vi "Format Library List Table.vi"(5 "Detail Level":T1, 7 "Msg Chain in":string, 8 "error in (no error)":errorcluster, 10 "Library Info Array":T2[](array[typedef]), 11 "VIDoc Printer - Confluence In":refnum<class "VIDoc Printer - Confluence.lvclass">) -> (0 "error out":errorcluster, 2 "Table Text":string, 3 "VIDoc Printer - Confluence Out":refnum<class "VIDoc Printer - Confluence.lvclass">)   [LabVIEW 2023, in "VIDoc Printer - Confluence.lvlib" / "VIDoc Printer - Confluence.lvclass"]
uses:
  VIDoc Printer - Confluence.lvclass
  C:/projects/DMC/Tooling/Git-Action-Service/Source/Documentation Generation/Printers/Printer/VIDoc Printer.lvclass
  Parsing/TypeDefs/Base Library Info Cluster.ctl
  <vilib>/picture/picture.llb/imagedata.ctl
  Settings/Printer Settings/Detail Level Enum.ctl
  VIDoc Printer - Confluence.lvclass/VIDoc Printer - Confluence.ctl
  Accessors/Get Library Column Ordering - Full.vi
  Accessors/Get Library Column Ordering - Minimal.vi
  Accessors/Get Library Column Ordering - Standard.vi
  Accessors/Get Sortable Tables.vi
  Printer/VIDoc Printer.lvclass
  UI Interaction/UI Interaction.lvclass
  Confluence Formatting/Confluence Formatting.lvlib
  C:/projects/DMC/Tooling/Git-Action-Service/Source/Documentation Generation/Printers/Confluence Printer/VIDoc Printer - Confluence.lvclass
  Parsing/VIDoc Parsing.lvlib
  Settings/Printer Settings/Printer Settings.lvclass
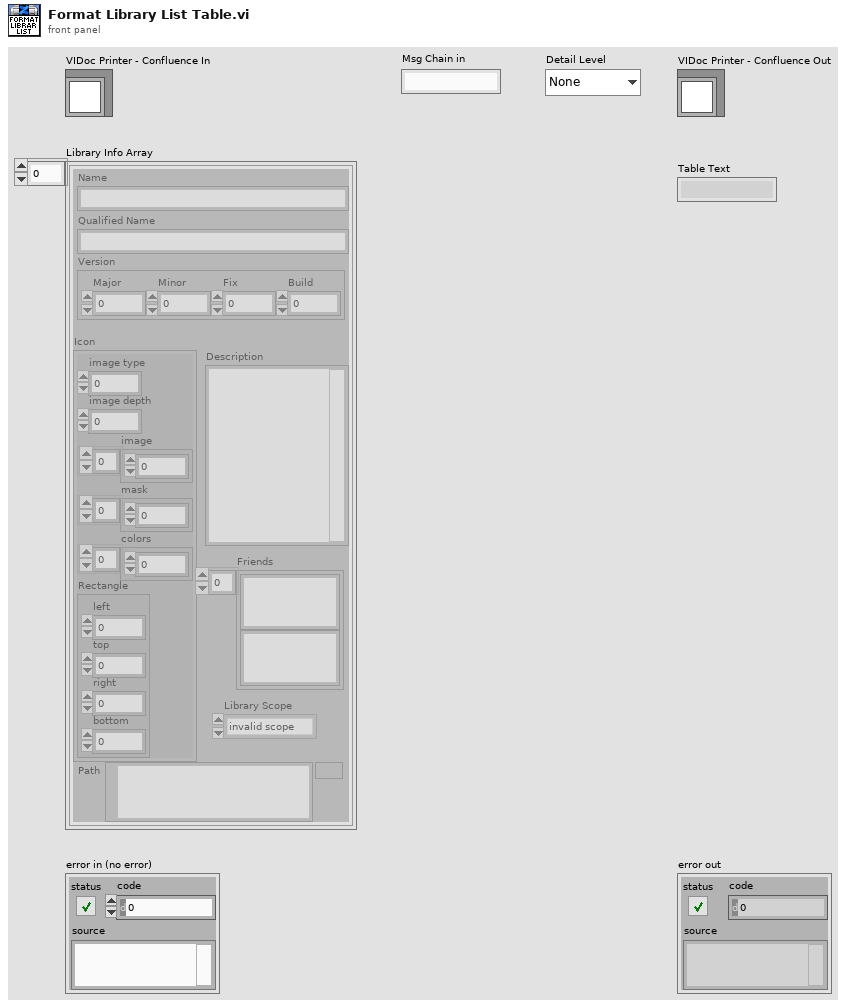
[diagram p1: front panel]
types:
  T1 = typedef "VIDoc Printer.lvlib/Printer Settings.lvclass/Detail Level Enum.ctl" = enum16{"None", "Minimal", "Standard", "Full"}
  T2 = typedef "VIDoc Parsing.lvlib/Base Library Info Cluster.ctl" = cluster{"Name":string, "Icon":T3, "Version":cluster{"Major":u16, "Minor":u16, "Fix":u16, "Build":u16}, "Description":string, "Path":path, "Friends":string[], "Library Scope":enum32{"invalid scope", "public", "private", "protected", "community"}, "Qualified Name":string}
  T3 = typedef "imagedata.ctl" = cluster{"image type":i32, "image depth":i32, "image":u8[], "mask":u8[], "colors":u32[], "Rectangle":cluster{"left":i16, "top":i16, "right":i16, "bottom":i16}}
  T4 = cluster{"Major":u16, "Minor":u16, "Fix":u16, "Build":u16}
  T5 = typedef "VIDoc Printer - Confluence.lvlib/VIDoc Settings - Confluence.lvclass/Class Info Column.ctl" = enum16{"Image", "Name", "Description", "Version", "Last Change", "Author", "Commit Hash", "Branch", "Qualified Name", "TransferMustOverrides", "ChildRefsRestricted"}
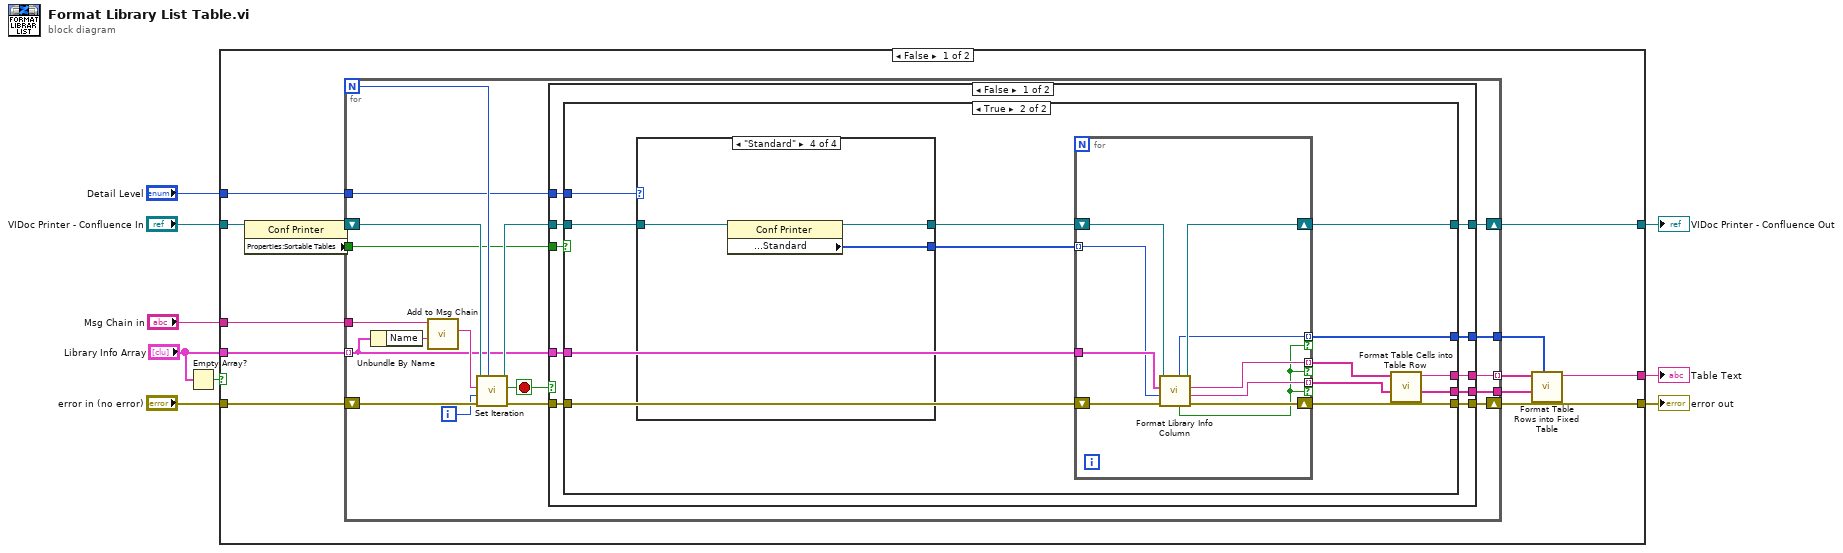
[diagram p0: block diagram]
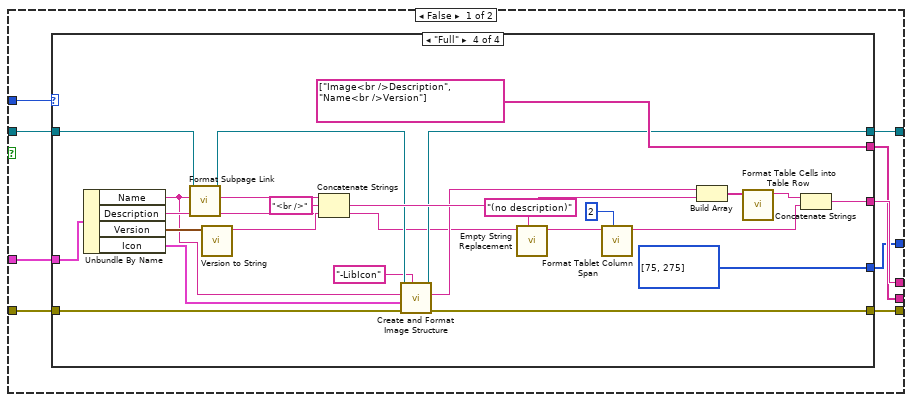
[diagram p2: hidden frame]
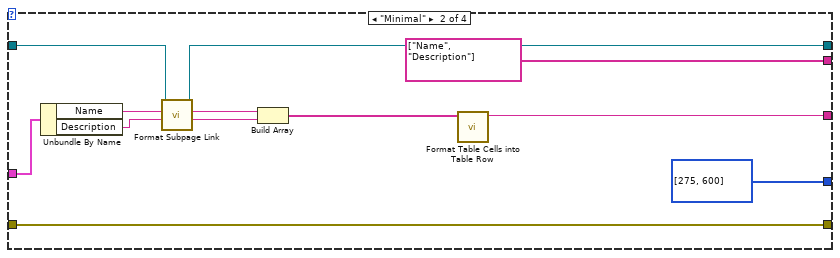
[diagram p4: hidden frame]
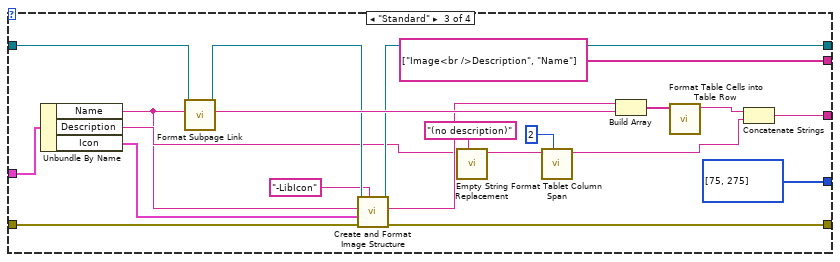
[diagram p5: hidden frame]
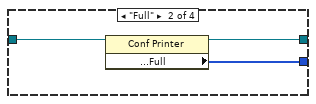
[diagram p7: hidden frame]
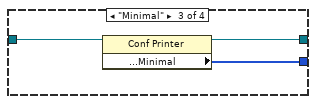
[diagram p8: hidden frame]
diagram:
  n1 = Empty Array?(array="Library Info Array") -> (empty?=w5:bool)
  n2 = case shown="False" w5 {
    tunnel: [w22 w153] -> w9
    tunnel: [w13 _] -> w8
    tunnel: [w21 w154] -> w7
    tunnel: "VIDoc Printer - Confluence In" -> [w17 w154]
    tunnel: "error in (no error)" -> [w20 w153]
    tunnel: "Library Info Array" -> [w19 _]
    tunnel: "Msg Chain in" -> [w18 _]
    tunnel: "Detail Level" -> [w16 _]
    frame False {
      n3 = property class="Conf Printer"(reference=w17) -> (reference out=w11:refnum<class "VIDoc Printer - Confluence.lvclass">, "Properties:Sortable Tables"=w10:bool)  [unwired: 1 in, 1 out]
      n4 = for {
        N -> [w38]
        shift-right: [w29] -> w22
        shift-left: w20 -> [w40]
        shift-right: [w31] -> w21
        shift-left: w11 -> [w39]
        tunnel: w19 -> [w26] mode=indexing
        tunnel: w18 -> [w34]
        tunnel: w16 -> [w30]
        tunnel: [w28] -> w15 mode=indexing
        tunnel: [w27] -> w14
        tunnel: [w25] -> w12
        tunnel: w10 -> [w23]
        i -> [w37]
        stop <- w24 stop-if-true
        n5 = Unbundle By Name(w26) -> ("Name"=w36:string)
        n6 = call "Add to Msg Chain.vi"("New"=w36, "Msg Chain in"=w34) -> ("Msg Chain out"=w35:string)  [unwired: 9 in]
        n7 = call "Set Iteration.vi"("Progress Max"=w38, "error in (no error)"=w40, "Progress Value"=w37, "Message (No Message Update)"=w35, "VIDoc Printer In"=w39) -> ("error out"=w33:errorcluster, "Abort?"=w24:bool, "VIDoc Printer Out"=w32:refnum<class "VIDoc Printer - Confluence.lvclass">)  [unwired: 4 in]
        n8 = case shown="False" w24 {
          tunnel: w33 -> [w49 w152]
          tunnel: w32 -> [w48 w151]
          tunnel: [w46 w151] -> w31
          tunnel: w30 -> [w41 _]
          tunnel: [w45 w152] -> w29
          tunnel: [w44 _] -> w28
          tunnel: [w43 _] -> w27
          tunnel: w26 -> [w47 _]
          tunnel: [w42 _] -> w25
          tunnel: w23 -> [w50 _]
          frame False {
            n9 = case shown="True" w50 {
              tunnel: w49 -> [w59 w129]
              tunnel: w48 -> [w57 w119]
              tunnel: w47 -> [w58 w123]
              tunnel: [w56 w126] -> w46
              tunnel: [w55 w124] -> w45
              tunnel: [w54 w130] -> w44
              tunnel: [w53 w128] -> w43
              tunnel: [w52 w125] -> w42
              tunnel: w41 -> [w51 w122]
              frame False {
                n10 = case shown="\"Full\"" w51 {
                  tunnel: [_ w68 w91 w116] -> w54
                  tunnel: [w61 w67 w86 w107] -> w55
                  tunnel: w59 -> [w61 w67 w75 w97]
                  tunnel: [w60 w63 w83 w103] -> w56
                  tunnel: w57 -> [w60 w62 w82 w106]
                  tunnel: w58 -> [_ w72 w92 w117]
                  tunnel: [_ string[] ["Name", "Description"] ("Table Headers") string[] ["Image<br />Description", "Name"] ("Table Headers") string[] ["Image<br />Description", "Name<br />Version"] ("Table Headers")] -> w53
                  tunnel: [_ i16[] [275, 600] ("Column Pixel Widths") i16[] [75, 275] ("Column Pixel Widths") i16[] [75, 275] ("Column Pixel Widths")] -> w52
                  frame "None" {
                  }
                  frame "Minimal" {
                    n11 = Unbundle By Name(w72) -> ("Name"=w71:string, "Description"=w70:string)
                    n12 = call "Format Subpage Link.vi"("Qualified Name"=w71, "VIDoc Printer - Confluence In"=w62) -> ("Linked HTML"=w64:string, "VIDoc Printer - Confluence Out"=w63:refnum<class "VIDoc Printer - Confluence.lvclass">)  [unwired: 7 in, 1 out]
                    n13 = Build Array(w64, w70) -> (w69:string[])
                    n14 = call "Format Table Cells into Table Row.vi"("Table Cells"=w69) -> ("Table Row Text"=w68:string)  [unwired: 10 in]
                  }
                  frame "Standard" {
                    n15 = Unbundle By Name(w92) -> ("Name"=w73:string, "Description"=w78:string, "Icon"=w74:T3)
                    n16 = call "Format Subpage Link.vi"("Qualified Name"=w73, "VIDoc Printer - Confluence In"=w82) -> ("Linked HTML"=w89:string, "VIDoc Printer - Confluence Out"=w84:refnum<class "VIDoc Printer - Confluence.lvclass">)  [unwired: 7 in, 1 out]
                    n17 = call "Create and Format Image Structure.vi"("Name Addition"="-LibIcon" ("string"), "Error in"=w75, "Image Data"=w74, "Name"=w73, "VIDoc Printer - Confluence In"=w84) -> ("Error out"=w86:errorcluster, "Image Structure Text"=w85:string, "VIDoc Printer - Confluence Out"=w83:refnum<class "VIDoc Printer - Confluence.lvclass">)  [unwired: 3 in, 1 out]
                    n18 = call "Empty String Replacement.vi"("Empty"="(no description)", "String"=w78) -> ("String Out"=w80:string)  [unwired: 9 in]
                    n19 = call "Format Tablet Column Span.vi"("Column Count"=2 ("Row Span (None)"), "Spanned Cell Text"=w80) -> ("Row Text"=w77:string)  [unwired: 9 in]
                    n20 = Build Array(w85, w89) -> (w88:string[])
                    n21 = call "Format Table Cells into Table Row.vi"("Table Cells"=w88) -> ("Table Row Text"=w87:string)  [unwired: 10 in]
                    n22 = Concatenate Strings(w87, w77) -> (w91:string)
                  }
                  frame "Full" {
                    n23 = Unbundle By Name(w117) -> ("Name"=w95:string, "Description"=w100:string, "Version"=w115:T4, "Icon"=w96:T3)
                    n24 = call "Format Subpage Link.vi"("Qualified Name"=w95, "VIDoc Printer - Confluence In"=w106) -> ("Linked HTML"=w113:string, "VIDoc Printer - Confluence Out"=w104:refnum<class "VIDoc Printer - Confluence.lvclass">)  [unwired: 7 in, 1 out]
                    n25 = call "Version to String.vi"("Version"=w115) -> ("String"=w114:string)  [unwired: 10 in]
                    n26 = Concatenate Strings(w113, "<br />" ("string"), w114) -> (w108:string)
                    n27 = call "Create and Format Image Structure.vi"("Name Addition"="-LibIcon" ("string"), "Error in"=w97, "Image Data"=w96, "Name"=w95, "VIDoc Printer - Confluence In"=w104) -> ("Error out"=w107:errorcluster, "Image Structure Text"=w105:string, "VIDoc Printer - Confluence Out"=w103:refnum<class "VIDoc Printer - Confluence.lvclass">)  [unwired: 3 in, 1 out]
                    n28 = call "Empty String Replacement.vi"("Empty"="(no description)", "String"=w100) -> ("String Out"=w101:string)  [unwired: 9 in]
                    n29 = call "Format Tablet Column Span.vi"("Column Count"=2 ("Row Span (None)"), "Spanned Cell Text"=w101) -> ("Row Text"=w98:string)  [unwired: 9 in]
                    n30 = Build Array(w105, w108) -> (w111:string[])
                    n31 = call "Format Table Cells into Table Row.vi"("Table Cells"=w111) -> ("Table Row Text"=w110:string)  [unwired: 10 in]
                    n32 = Concatenate Strings(w110, w98) -> (w116:string)
                  }
                }
              }
              frame True {
                n33 = case shown="\"Standard\"" w122 {
                  tunnel: [_ w132 w135 w138] -> w121
                  tunnel: [w131 w133 w136 w139] -> w120
                  tunnel: w119 -> [w131 w134 w137 w140]
                  frame "None" {
                  }
                  frame "Full" {
                    n34 = property class="Conf Printer"(reference=w134) -> (reference out=w133:refnum<class "VIDoc Printer - Confluence.lvclass">, "Properties:Table Column Ordering:Library:Full"=w132:T5[])  [unwired: 1 in, 1 out]
                  }
                  frame "Minimal" {
                    n35 = property class="Conf Printer"(reference=w137) -> (reference out=w136:refnum<class "VIDoc Printer - Confluence.lvclass">, "Properties:Table Column Ordering:Library:Minimal"=w135:T5[])  [unwired: 1 in, 1 out]
                  }
                  frame "Standard" {
                    n36 = property class="Conf Printer"(reference=w140) -> (reference out=w139:refnum<class "VIDoc Printer - Confluence.lvclass">, "Properties:Table Column Ordering:Library:Standard"=w138:T5[])  [unwired: 1 in, 1 out]
                  }
                }
                n37 = for {
                  shift-right: [w149] -> w124
                  shift-left: w129 -> [w150]
                  tunnel: [w148] -> w128 mode=indexing if=w141
                  tunnel: [w147] -> w127 mode=indexing if=w141
                  shift-right: [w145] -> w126
                  shift-left: w120 -> [w146]
                  tunnel: [w144] -> w125 mode=indexing if=w141
                  tunnel: w123 -> [w143]
                  tunnel: w121 -> [w142] mode=indexing
                  n38 = call "Format Library Info Column.vi"("error in (no error)"=w150, "Column"=w142, "Library Info"=w143, "VIDoc Printer - Confluence In"=w146) -> ("error out"=w149:errorcluster, "Header"=w148:string, "Cell Text"=w147:string, "VIDoc Printer - Confluence Out"=w145:refnum<class "VIDoc Printer - Confluence.lvclass">, "Viable Value?"=w141:bool, "Pixel Width"=w144:i16)  [unwired: 2 in]
                }
                n39 = call "Format Table Cells into Table Row.vi"("Table Cells"=w127) -> ("Table Row Text"=w130:string)  [unwired: 10 in]
              }
            }
          }
          frame True {
          }
        }
      }
      n40 = call "Format Table Rows into Fixed Table.vi"("Column Pixel Widths"=w12, "Table Headers"=w14, "Table Rows"=w15) -> ("Table Text"=w13:string)  [unwired: 8 in]
    }
    frame True {
    }
  }
  "error out" <- w9
  "Table Text" <- w8
  "VIDoc Printer - Confluence Out" <- w7
